vi "Configure Standard Waveform.vi"   [LabVIEW 2012, in "RIGOL DG4000 Series.lvlib"]
doc: "Select a standard waveform and configure the frequency/sample rate, amplitude, offset, and phase for it.\nStandard waveform includes Custom, Harmonic, Noise, Pulse, Ramp, Sine, Square."
uses:
  <instrlib>/RIGOL DG4000 Series/RIGOL DG4000 Series.lvlib
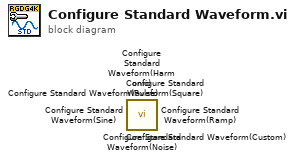
[diagram p0: block diagram]
diagram:
  n1 = call <instrlib>:"Configure Standard Waveform(Noise).vi"() -> ()  [unwired: 14 in, 2 out]
  n2 = call <instrlib>:"Configure Standard Waveform(Square).vi"() -> ()  [unwired: 14 in, 2 out]
  n3 = call <instrlib>:"Configure Standard Waveform(Sine).vi"() -> ()  [unwired: 14 in, 2 out]
  n4 = call <instrlib>:"Configure Standard Waveform(Ramp).vi"() -> ()  [unwired: 14 in, 2 out]
  n5 = call <instrlib>:"Configure Standard Waveform(Pulse).vi"() -> ()  [unwired: 14 in, 2 out]
  n6 = call <instrlib>:"Configure Standard Waveform(Harmonic).vi"() -> ()  [unwired: 14 in, 2 out]
  n7 = call <instrlib>:"Configure Standard Waveform(Custom).vi"() -> ()  [unwired: 14 in, 2 out]
